vi "Generation Stream Control (IQ 1 SPC).vi"(0 "data in":T2, 1 "input valid":bool, 2 "request state":T1, 3 "num samples":u64, 4 "initial padding":u64, 5 "final padding":u64, 7 "ready for output (T)":bool=TRUE, 8 "reset":bool, 9 "start trigger":bool) -> (11 "ready for start":bool, 12 "metadata":u64, 13 "ready for input":bool, 14 "data out":T2, 15 "output valid":bool, 16 "actual state":T1, 17 "samples transferred":u64)   [LabVIEW 2018, in "Streaming FPGA.lvlib"]
doc: "<B>General</B>\n\nThis VI controls the signal generation data flow with a state machine controller. This enables the control and monitoring of finite and continuous streams of data between nodes using 4-wire handshaking.\n\n<B>Signals</B>\n\nThe stream is controlled by the <B>request state</B>, <B>num samples</B>, <B>initial padding</B>, <B>final padding</B> and <B>start trigger</B> inputs. The stream is monitored by the <B>actual state</B>, <B>ready for start</B> and <B>samples transferred</B> outputs. In addition, <b>metadata</b> is available for publishing details about the form/function of the stream.\n\nThe upstream node can provide data on the <B>data in</B> input by setting the <B>input valid</B> input to true. The data provided on the <B>data in</B> input is accepted if the <B>input valid</B> input is true and the <B>ready for input</B> output was true in the previous cycle. If the <B>ready for input</B> output was false in the previous cycle, then the <B>data in</B> and <B>input valid</B> inputs are ignored in the current cycle.\n\nThe <B>output valid</B> output is set to true when data is available on the <B>data out</B> output. The downstream node should set the <B>ready for output</B> input to true when it is ready for data. If the <B>ready for output</B> input is true and the <B>output valid</B> output is also true, then the downstream node should accept the data provided on the <B>data out</B> output. If the <B>ready for output</B> input is false or if the <B>output valid</B> output is false, then the downstream should ignore the <B>data out</B> output.\n\n<B>Detailed Operation</B>\n\nThere are two signal generation modes: finite or continuous mode. Each time a signal generation is started <B>initial padding</B> number of padding samples are provided to the downstream node first, followed by <B>num samples</B> samples (in case of finite mode) or an unspecified number of samples (in case of continuous mode) provided by the upstream node. At the end of the signal generation <B>final padding</B> number of padding samples are provided to the downstream node. A finite signal generation can be started by transitioning the state machine from the Idle state to the Finite Transfer state. A continuous signal generation can be started by transitioning the state machine from the Idle state to the Continuous state. Transitioning from the Idle state to the Finite Transfer or Continuous state does not start the signal generation immediately, when transitioning into these states the state machine always waits for a start trigger before starting the generation. The state machine sets the <B>ready for start</B> output to true when it is waiting for a start trigger in the next cycle (otherwise this output is false), the start trigger can be provided on the <B>start trigger</B> input by setting this input to true. The <B>start trigger</B> to <B>output valid</B> delay is 1 cycle. Note that this VI assumes that the signal generation should be continuous: during the signal generation if the <B>ready for output</B> input is true, but no data can be provided to the downstream node, the state machine aborts the signal generation and enters the Error state.\n\n<B>samples transferred</B> is updated with the number of upstream node provided samples accepted by the downstream node in the current cycle, that is, this counter does not include the number of initial/final padding samples provided to the downstream node.\n\nIn finite mode the state machine enters the Done state once the signal generation is finished. In the Done state the samples transferred continues to be reported until the user requests that the state machine return to Idle. A signal generation can be aborted by entering the Cancel state. When entering the Cancel state, the final padding samples are still provided to the downstream node (in case the generation was started), then the state machine transitions to the Not Ready state, then it can transition into the Idle state.\n\nThis node uses an internal cache for storing samples provided by the upstream node. The upstream node is read in advance, samples stored in the internal cache are not flushed when a generation finishes, the samples remaining in the cache are returned during the next signal generation. The cache can be cleared by setting the <B>reset</B> input to true. This will also abort any ongoing signal generations but does not change the state of the internal state machine. In order to completely reset this VI set the <B>request state</B> input to Idle, set the <B>reset</B> input to true, wait until the <B>actual state</B> output indicates Idle, then set the <B>reset</B> input to false. Note that the upstream node is not read while this VI is in the Idle state.\n\n<b>States</b>\n\nThere are seven potential states for a stream defined by the Stream State.ctl typedef. All commanded states should be monitored from the controlling loop if it is important to ensure that the state is actually entered. The <B>request state</B> commands the stream into a state, and <B>actual state</B> reflects the current actual state.\n\nIdle - when the stream is ready to enter into an active state, it is in the Idle state. While it can be commanded directly to Idle from any state, it is advisable to do so with caution as samples abandoned in transfers may still need to be manually cleared out. It is generally safe to go directly from Done to Idle, and it is generally safe to request a transition from Not Ready to Idle. Other states may require further clean-up such as stopping/starting FIFOs or resetting other code under the command of the stream. Consider using Cancel instead (such as through the \"Stop Stream.vi\" in the host environment). While in Idle, <B>samples transferred</B> is reset to 0. \n\nFinite Transfer - Execute a transfer for the requested number of samples. Upon an orderly completion, this VI will automatically enter the Done state. If a stream underflows because the <B>ready for output</B> input is true, but no data can be provided to the downstream node, then the state machine enters the Error state.\n\nContinuous - Execute a transfer indefinitely. This state operates identically to the Finite Transfer state, but without regard to the <B>num samples</B> input.\n\nDone - In an orderly termination of a finite stream, the stream should end up here. At this point, <B>samples transferred</B> accurately reflects the terminal state of the transfer. The Done state should be exited by requesting Idle. Further active transfer modes (Finite or Continuous) will be ignored. This allows the host to distinguish between streams that are prematurely terminated (thus potentially requiring a flush of abandoned data) and ones that completed naturally.\n\nError - If the stream detects an unplanned interruption of the data, it enters the Error state. The only way to exit the Error state is to command the Generation Stream Control to Idle or Not Ready. When commanded to Idle or Not Ready, the Generation Stream Control advances first to Not Ready after the final padding samples are provided to the downstream node.\n\nNot Ready - In this state, the Generation Stream Control remains in the Not Ready state until the final padding samples are provided to the downstream node and the Generation Stream Control is commanded to Idle. This prevents starting a transfer in an obviously invalid state, and allows host control to wait until the not ready state is removed (such as by clearing out a FIFO under the streaming API's control).\n\nCancel - This state is indistinguishable from Error, but allows the controlling VI to know what condition caused the transfer to terminate."
uses:
  Streaming FPGA.lvlib
  <instrlib>/_niInstr/DSP/v1/Shared/Public/IQ Data.ctl
  <instrlib>/_niInstr/Streaming/v1/Common/Stream State.ctl
  <instrlib>/_niInstr/DSP/v1/Shared/niInstr DSP v1 Shared.lvlib
  <instrlib>/_niInstr/Streaming/v1/Common/niInstr Streaming v1 Common.lvlib
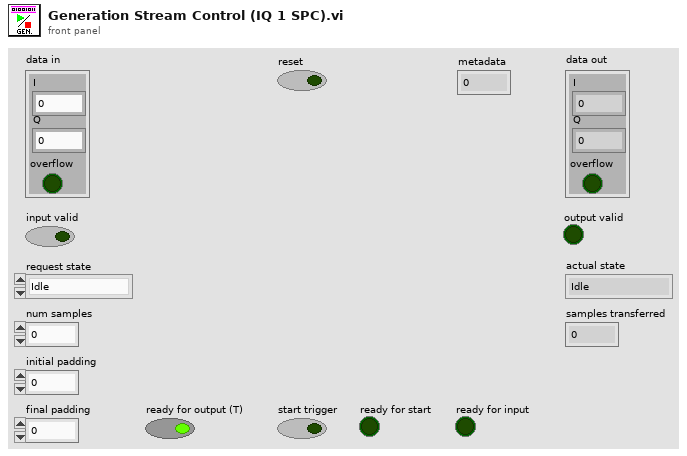
[diagram p1: front panel]
types:
  T1 = typedef "niInstr Streaming v1 Common.lvlib/Stream State.ctl" = enum8{"Idle", "Finite Transfer", "Continuous", "Done", "Error", "Not Ready", "Cancel"}
  T2 = typedef "niInstr DSP v1 Shared.lvlib/IQ Data.ctl" = cluster{"I":fxp<+/-,18,1>, "Q":fxp<+/-,18,1>, "overflow":bool}
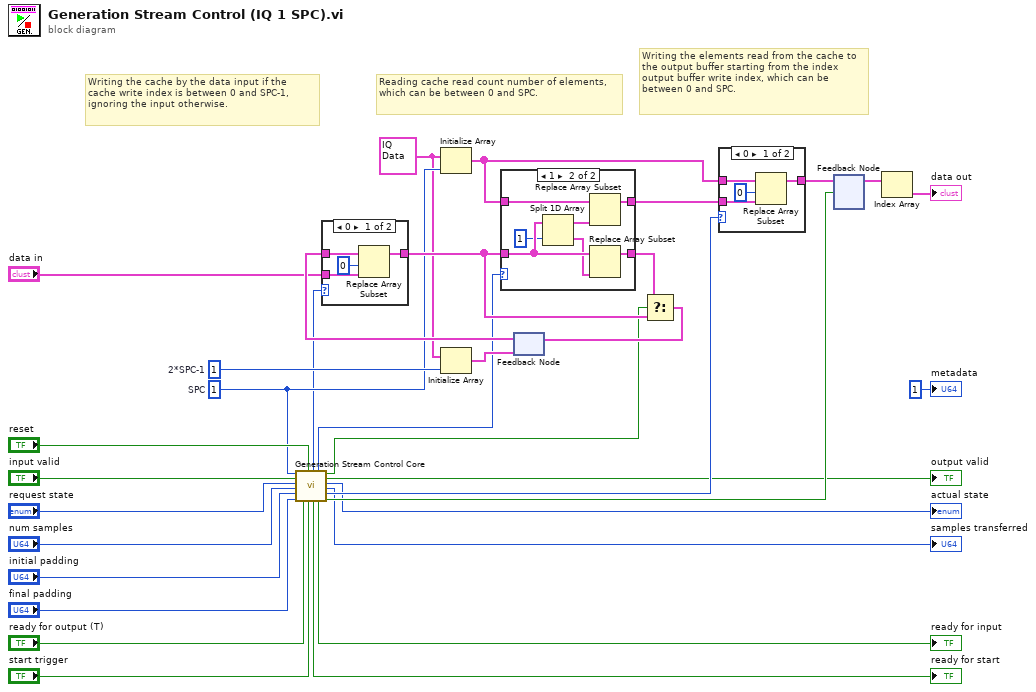
[diagram p0: block diagram]
diagram:
  w1 = T2 {"I"=0.0, "Q"=0.0, "overflow"=FALSE}
  w22 = u8 1  # SPC
  w32 = u8 1  # 2*SPC-1
  # "Writing the elements read from the cache to the output buffer starting from the index output buffer write index, which can be between 0 and SPC."
  # "Reading cache read count number of elements, which can be between 0 and SPC."
  # "Writing the cache by the data input if the cache write index is between 0 and SPC-1, ignoring the input otherwise."
  n1 = call "Generation Stream Control Core.vi"("SPC"=w22, "input valid"="input valid", "request state"="request state", "num samples"="num samples", "initial padding"="initial padding", "final padding"="final padding", "ready for output (T)"="ready for output (T)", "reset"="reset", "start trigger"="start trigger") -> ("cache write index"=w21:u8, "ready for start"=→"ready for start":bool, "cache read count"=w20:u8, "ready for input"=→"ready for input":bool, "cache discard read elements"=w19:bool, "output valid"=→"output valid":bool, "actual state"=→"actual state":T1, "samples transferred"=→"samples transferred":u64, "output buffer write index"=w18:u8, "output buffer latch enable"=w17:bool)  [unwired: 1 in]
  n2 = Initialize Array(w1, w22) -> (w10:T2[])
  n3 = Initialize Array(w1, w32) -> (w31:T2[])
  n4 = feedback #1(w31) -> (w33:T2[])
  n5 = case shown="0" w21 {
    tunnel: w33 -> [w37 w38]
    tunnel: "data in" -> [w36 _]
    tunnel: [w34 w38] -> w25
    frame 0 {
      n6 = Replace Array Subset(array=w37, new element=w36, index=0) -> (w34:T2[])
    }
    frame Default {
    }
  }
  n7 = case shown="1" w20 {
    tunnel: w25 -> [w39 w47]
    tunnel: [w39 w42] -> w27
    tunnel: w10 -> [w40 w45]
    tunnel: [w40 w43] -> w29
    frame 0, Default {
    }
    frame 1 {
      n8 = Split 1D Array(array=w47, index=1) -> (first subarray=w44:T2[], second subarray=w46:T2[])
      n9 = Replace Array Subset(array=w45, new element=w44) -> (w43:T2[])  [unwired: 1 in]
      n10 = Replace Array Subset(array=w47, new element=w46) -> (w42:T2[])  [unwired: 1 in]
    }
  }
  n11 = Select(t=w27, s=w19, f=w25) -> (s? t:f=w26:T2[])
  n12 = feedback-in #1(w26) -> ()
  n13 = case shown="0" w18 {
    tunnel: w10 -> [w51 w52]
    tunnel: w29 -> [w50 _]
    tunnel: [w48 w52] -> w28
    frame 0 {
      n14 = Replace Array Subset(array=w51, new element=w50, index=0) -> (w48:T2[])
    }
    frame 1, Default {
    }
  }
  n15 = feedback-in #2(w28, w17) -> ()
  n16 = feedback #2() -> (w4:T2[])  [unwired: 1 in]
  n17 = Index Array(array=w4) -> (element=→"data out":T2)  [unwired: 1 in]
  "metadata" <- u64 1 ("metadata")
